vi "saveLastId.vi"(1 "lastId":string, 2 "path":path) -> ()   [LabVIEW 2010]
uses:
  <vilib>/Utility/config.llb/Write Key (String).vi
  <vilib>/Utility/config.llb/NI_LVConfig.lvlib
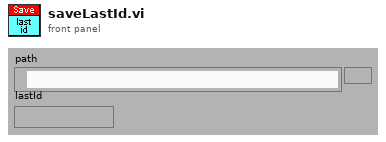
[diagram p1: front panel]
types:
  T1 = typedef "NI_LVConfig.lvlib/Config Data RefNum.ctl" = refnum<k1>
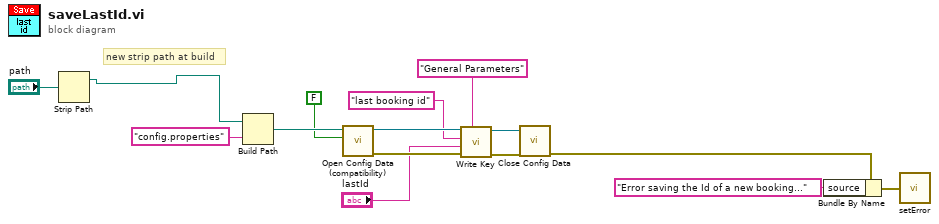
[diagram p0: block diagram]
diagram:
  # "new strip path at build"
  n1 = Strip Path(path="path") -> (stripped path=w1:path)  [unwired: 1 out]
  n2 = Build Path(base path=w1, name or relative path="config.properties") -> (appended path=w13:path)
  n3 = call <vilib>:"Open Config Data (compatibility).vi"("create file if necessary (T)"=FALSE ("create file if necessary? (T)"), "configuration file path"=w13) -> ("error out"=w10:errorcluster, "refnum"=w11:T1)  [unwired: 7 in, 1 out]
  n4 = call-poly <vilib>:"Write Key.vi"("section"="General Parameters", "error in (no error)"=w10, "value"="lastId", "key"="last booking id", "refnum"=w11) -> ("error out"=w5:errorcluster, "refnum out"=w6:T1)  [unwired: 1 in, 4 out]
  n5 = call <vilib>:"Close Config Data.vi"("error in (no error)"=w5, "refnum"=w6) -> ("error out"=w4:errorcluster)  [unwired: 1 in, 8 out]
  n6 = Bundle By Name(cluster=w4, "source"="Error saving the Id of a new booking...") -> (w2:errorcluster)
  n7 = call "setError.vi"("error"=w2) -> ()  [unwired: 1 out]
